vi "SingleAcquisition.vi"() -> ()   [LabVIEW 2018]
uses:
  D:/SVN/PM/sdk/AppSamples/LabVIEWSamples/trunk/Release/2018/Dependencies/PVCamNET.dll
  Dependencies/PVCamNET.dll
panel:
  in  "?":bool
  in  "Exposure time":dbl=30.0
  in  "?":bool
  # "SingleAcquisition.vi\n\nDescription:\nThis sample code lets the user use single acqusition mode\nwith the user's preferred exposure time. \n\nSteps to run:\n1. Click \"Run\"\n2. Enter exposure time\n3. Click \"START\"\n4. Click \"STOP\""
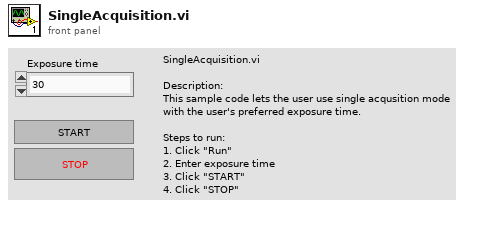
[diagram p1: front panel]
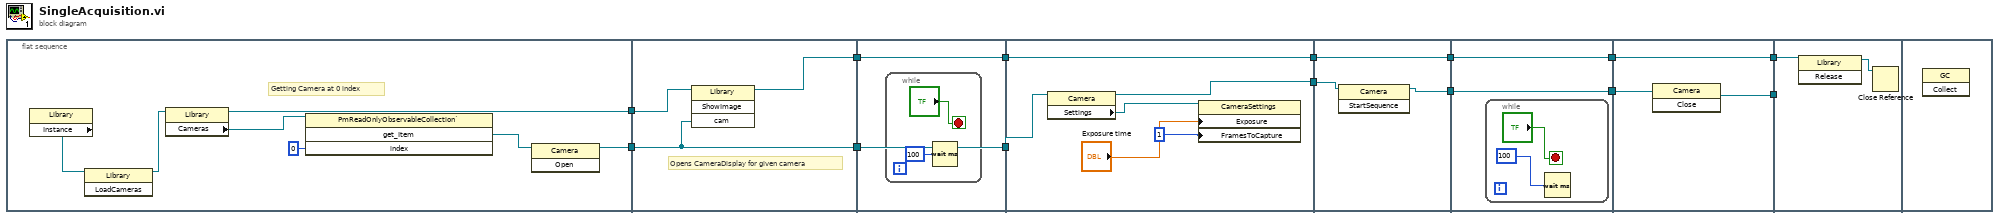
[diagram p0: block diagram]
diagram:
  n1 = flat-sequence {
    tunnel: [w17] -> w14
    tunnel: [w18] -> w13
    tunnel: w14 -> [w24]
    tunnel: w13 -> [w23]
    tunnel: [w23] -> w12
    tunnel: [w22] -> w11
    tunnel: w12 -> [w26]
    tunnel: [w26] -> w9
    tunnel: w11 -> [w25]
    tunnel: [w25] -> w10
    tunnel: [w34] -> w8
    tunnel: [w33] -> w7
    tunnel: w10 -> [w33]
    tunnel: w9 -> [w32]
    tunnel: w8 -> [w36]
    tunnel: [w35] -> w6
    tunnel: [w37] -> w5
    tunnel: w7 -> [w37]
    tunnel: w6 -> [w39]
    tunnel: [w39] -> w2
    tunnel: [w38] -> w1
    tunnel: w5 -> [w38]
    tunnel: w2 -> [w44]
    tunnel: w1 -> [w42]
    tunnel: [w43] -> w4
    tunnel: [w42] -> w3
    tunnel: w4 -> [_]
    tunnel: w3 -> [w46]
    frame #0 {
      # "Getting Camera at 0 index"
      n2 = property class="Library"() -> ("Instance"=w16:refnum<k24>)  [unwired: 2 in, 2 out]
      n3 = invoke class="Library" method="LoadCameras"(reference=w16) -> (reference out=w15:refnum<k24>)  [unwired: 2 in, 2 out]
      n4 = property class="Library"(reference=w15) -> (reference out=w17:refnum<k24>, "Cameras"=w21:refnum<k24>)  [unwired: 1 in, 1 out]
      n5 = invoke class="PmReadOnlyObservableCollection`" method="get_Item"(reference=w21, "index"=0) -> ("get_Item"=w19:refnum<k24>)  [unwired: 2 in, 3 out]
      n6 = invoke class="Camera" method="Open"(reference=w19) -> (reference out=w18:refnum<k24>)  [unwired: 2 in, 2 out]
    }
    frame #1 {
      # "Opens CameraDisplay for given camera"
      n7 = invoke class="Library" method="ShowImage"(reference=w24, "cam"=w23) -> (reference out=w22:refnum<k24>)  [unwired: 2 in, 3 out]
    }
    frame #2 {
      n8 = while {
        stop <- "?" stop-if-true
        n9 = Wait (ms)(milliseconds to wait=u32 100) -> ()  [unwired: 1 out]
      }
    }
    frame #3 {
      n10 = property class="Camera"(reference=w32) -> (reference out=w34:refnum<k24>, "Settings"=w29:refnum<k24>)  [unwired: 1 in, 1 out]
      n11 = property class="CameraSettings"(reference=w29, "Exposure"="Exposure time", "FramesToCapture"=u16 1) -> ()  [unwired: 1 in, 2 out]
    }
    frame #4 {
      n12 = invoke class="Camera" method="StartSequence"(reference=w36) -> (reference out=w35:refnum<k24>)  [unwired: 2 in, 2 out]
    }
    frame #5 {
      n13 = while {
        stop <- "?" stop-if-true
        n14 = Wait (ms)(milliseconds to wait=u32 100) -> ()  [unwired: 1 out]
      }
    }
    frame #6 {
      n15 = invoke class="Camera" method="Close"(reference=w44) -> (reference out=w43:refnum<k24>)  [unwired: 2 in, 2 out]
    }
    frame #7 {
      n16 = invoke class="Library" method="Release"(reference=w46) -> (reference out=w45:refnum<k24>)  [unwired: 2 in, 2 out]
      n17 = Close Reference(reference=w45) -> ()  [unwired: 1 in, 1 out]
    }
    frame #8 {
      n18 = invoke class="GC" method="Collect"() -> ()  [unwired: 3 in, 3 out]
    }
  }
